vi "Beam_Status.vi"() -> ()   [LabVIEW 2018]
panel:
  out "?":bool
  out "?":bool
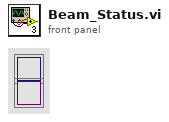
[diagram p1: front panel]
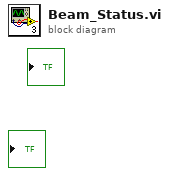
[diagram p0: block diagram]
diagram:
